vi "Ignore Items.vi"(8 "error in":errorcluster, 10 "extensions to filter, separated by comma":string, 11 "Tree":refnum<vi>) -> (0 "error out":errorcluster)   [LabVIEW 2020, in "LV Project Items Parser.lvlib"]
uses:
  LV Project Items Parser.lvlib
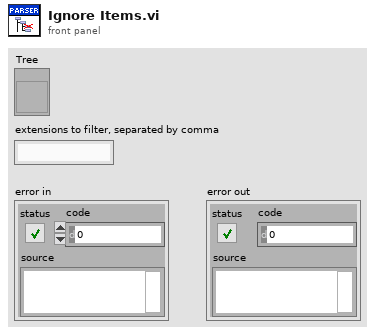
[diagram p1: front panel]
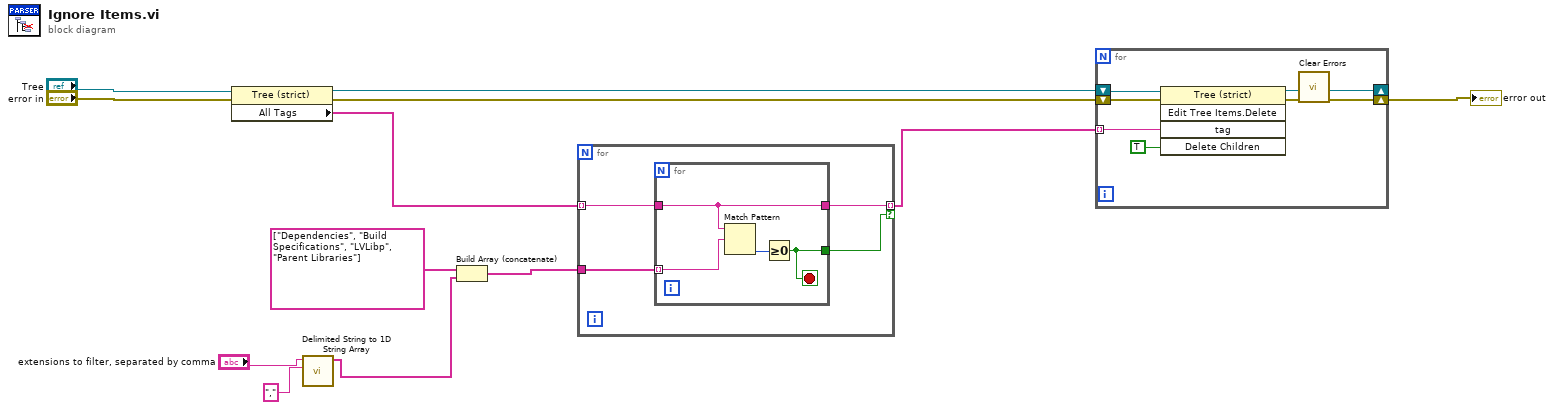
[diagram p0: block diagram]
diagram:
  n1 = property class="Tree (strict)"(reference="Tree", error in="error in") -> (reference out=w8:refnum<vi>, error out=w9:errorcluster, "All Tags"=w7:string[])
  n2 = call <vilib>:"Delimited String to 1D String Array.vi"("delimiter"=",", "delimited string"="extensions to filter, separated by comma") -> ("string array"=w2:string[])  [unwired: 9 in]
  n3 = Build Array (concatenate)(string[] ["Dependencies", "Build Specifications", "LVLibp", "Parent Libraries"] ("Tag"), w2) -> (w4:string[])
  n4 = for {
    tunnel: w7 -> [w15] mode=indexing
    tunnel: w4 -> [w16]
    tunnel: [w14] -> w5 mode=indexing if=w13
    n5 = for {
      tunnel: w16 -> [w20] mode=indexing
      tunnel: w15 -> [w18]
      tunnel: [w17] -> w13
      tunnel: [w18] -> w14
      stop <- w17 stop-if-true
      n6 = Match Pattern(string=w18, regular expression=w20) -> (offset past match=w19:i32)  [unwired: 1 in, 3 out]
      n7 = Greater Or Equal To 0?(x=w19) -> (x >= 0?=w17:bool)
    }
  }
  n8 = for {
    tunnel: w5 -> [w25] mode=indexing
    shift-right: [w21] -> w12
    shift-left: w9 -> [w27]
    shift-right: [w22] -> _
    shift-left: w8 -> [w23]
    n9 = invoke on="Invoke Node" class="Tree (strict)" method="Edit Tree Items.Delete"(reference=w23, error in=w27, "tag"=w25, "Delete Children"=TRUE ("Delete Children?")) -> (reference out=w22:refnum<vi>, error out=w26:errorcluster)  [unwired: 1 in, 3 out]
    n10 = call <vilib>:"Clear Errors.vi"("error in (no error)"=w26) -> ("error out"=w21:errorcluster)  [unwired: 5 in, 1 out]
  }
  "error out" <- w12
